vi "R5DOControl.vi"(8 "error constant":errorcluster, 11 "LabVIEW Web Service":refnum<class "Web Service.lvclass">) -> ()   [LabVIEW 2016]
uses:
  <vilib>/wsapi/Web Service.lvclass
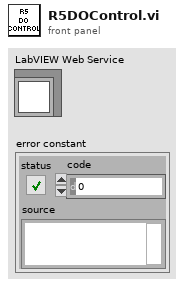
[diagram p1: front panel]
types:
  T1 = cluster{"Set Point, mg/L":dbl, "Tolerance, mg/L":dbl, "N2 Valve Gain":dbl, "Air Valve Gain":dbl}
  T2 = cluster{"Signal, mA":dbl, "Value, UNITS HERE":dbl}
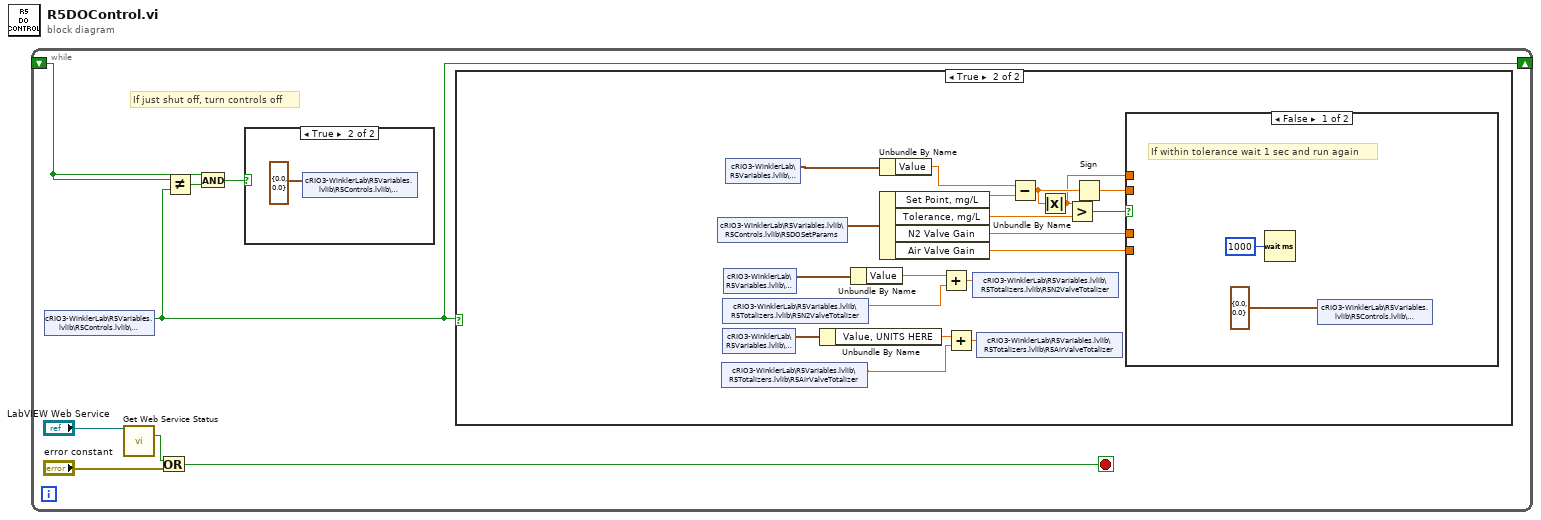
[diagram p0: block diagram]
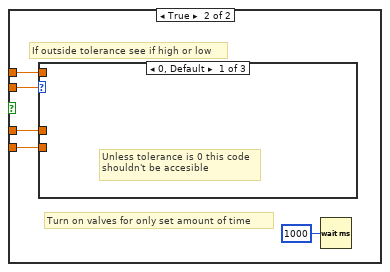
[diagram p4: hidden frame]
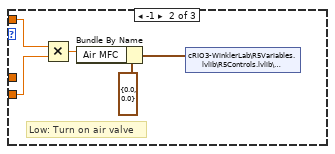
[diagram p5: hidden frame]
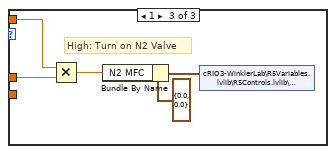
[diagram p6: hidden frame]
diagram:
  n1 = while {
    shift-right: [w1] -> _
    shift-left: _ -> [w2]
    stop <- w5 stop-if-true
    # "If just shut off, turn controls off"
    n2 = shared-variable "cRIO3-WinklerLab\\R5Variables.lvlib\\R5Controls.lvlib\\R5DOSwitch"() -> (w1:bool)  [unwired: 1 in, 1 out]
    n3 = call <vilib>:"Get Web Service Status.vi"("LabVIEW Web Service"="LabVIEW Web Service") -> ("service stopping?"=w8:bool)  [unwired: 12 in, 2 out]
    n4 = Or(x=w8, y="error constant") -> (x .or. y?=w5:bool)
    n5 = Not Equal?(x=w2, y=w1) -> (x != y?=w3:bool)
    n6 = And(x=w2, y=w3) -> (x .and. y?=w4:bool)
    n7 = case shown="True" w4 {
      frame False {
      }
      frame True {
        n8 = shared-variable "cRIO3-WinklerLab\\R5Variables.lvlib\\R5Controls.lvlib\\R5DOManual"(cluster{"Air MFC":dbl, "N2 MFC":dbl} {"Air MFC"=0.0, "N2 MFC"=0.0} ("R1DOManual")) -> ()  [unwired: 1 in, 1 out]
      }
    }
    n9 = case shown="True" w1 {
      frame False {
        # "Don't do anything if control is off"
      }
      frame True {
        n10 = shared-variable "cRIO3-WinklerLab\\R5Variables.lvlib\\R5Controls.lvlib\\R5DOSetParams"() -> (w16:T1)  [unwired: 1 in, 1 out]
        n11 = shared-variable "cRIO3-WinklerLab\\R5Variables.lvlib\\R5Totalizers.lvlib\\R5AirValveTotalizer"() -> (w13:dbl)  [unwired: 1 in, 1 out]
        n12 = shared-variable "cRIO3-WinklerLab\\R5Variables.lvlib\\R5Totalizers.lvlib\\R5N2ValveTotalizer"() -> (w12:dbl)  [unwired: 1 in, 1 out]
        n13 = shared-variable "cRIO3-WinklerLab\\R5Variables.lvlib\\R5Signals.lvlib\\R5Air"() -> (w14:T2)  [unwired: 1 in, 1 out]
        n14 = shared-variable "cRIO3-WinklerLab\\R5Variables.lvlib\\R5Signals.lvlib\\R5N2"() -> (w15:cluster{"Signal":dbl, "Value":dbl})  [unwired: 1 in, 1 out]
        n15 = shared-variable "cRIO3-WinklerLab\\R5Variables.lvlib\\R5Signals.lvlib\\R5DO"() -> (w17:cluster{"Signal":dbl, "Value":dbl})  [unwired: 1 in, 1 out]
        n16 = Unbundle By Name(w14) -> ("Value, UNITS HERE"=w19:dbl)
        n17 = Unbundle By Name(w15) -> ("Value"=w18:dbl)
        n18 = Unbundle By Name(w17) -> ("Value"=w28:dbl)
        n19 = Unbundle By Name(w16) -> ("Set Point, mg/L"=w27:dbl, "Tolerance, mg/L"=w26:dbl, "N2 Valve Gain"=w23:dbl, "Air Valve Gain"=w22:dbl)
        n20 = Add(x=w18, y=w12) -> (x+y=w11:dbl)
        n21 = Add(x=w19, y=w13) -> (x+y=w10:dbl)
        n22 = shared-variable "cRIO3-WinklerLab\\R5Variables.lvlib\\R5Totalizers.lvlib\\R5N2ValveTotalizer"(w11) -> ()  [unwired: 1 in, 1 out]
        n23 = shared-variable "cRIO3-WinklerLab\\R5Variables.lvlib\\R5Totalizers.lvlib\\R5AirValveTotalizer"(w10) -> ()  [unwired: 1 in, 1 out]
        n24 = Subtract(x=w28, y=w27) -> (x-y=w21:dbl)
        n25 = Absolute Value(x=w21) -> (abs(x)=w20:dbl)
        n26 = Greater?(x=w20, y=w26) -> (0:w25:bool)
        n27 = Sign(1:w21) -> (0:w24:dbl)
        n28 = case shown="False" w25 {
          tunnel: w24 -> [_ w35]
          tunnel: w23 -> [_ w34]
          tunnel: w22 -> [_ w33]
          tunnel: w20 -> [_ w32]
          frame False {
            # "If within tolerance wait 1 sec and run again"
            n29 = Wait (ms)(milliseconds to wait=u32 1000) -> ()  [unwired: 1 out]
            n30 = shared-variable "cRIO3-WinklerLab\\R5Variables.lvlib\\R5Controls.lvlib\\R5DOManual"(cluster{"Air MFC":dbl, "N2 MFC":dbl} {"Air MFC"=0.0, "N2 MFC"=0.0} ("R1DOManual")) -> ()  [unwired: 1 in, 1 out]
          }
          frame True {
            # "Turn on valves for only set amount of time"
            # "If outside tolerance see if high or low"
            n31 = case shown="0, Default" w35 {
              tunnel: w33 -> [_ w37 _]
              tunnel: w34 -> [_ _ w43]
              tunnel: w32 -> [_ w38 w44]
              frame 0, Default {
                # "Unless tolerance is 0 this code\nshouldn't be accesible"
              }
              frame -1 {
                # "Low: Turn on air valve"
                n32 = Multiply(x=w38, y=w37) -> (x*y=w39:dbl)
                n33 = Bundle By Name(cluster=cluster{"Air MFC":dbl, "N2 MFC":dbl} {"Air MFC"=0.0, "N2 MFC"=0.0} ("R1DOManual"), "Air MFC"=w39) -> (w36:cluster{"Air MFC":dbl, "N2 MFC":dbl})
                n34 = shared-variable "cRIO3-WinklerLab\\R5Variables.lvlib\\R5Controls.lvlib\\R5DOManual"(w36) -> ()  [unwired: 1 in, 1 out]
              }
              frame 1 {
                # "High: Turn on N2 Valve"
                n35 = Multiply(x=w44, y=w43) -> (x*y=w42:dbl)
                n36 = Bundle By Name(cluster=cluster{"Air MFC":dbl, "N2 MFC":dbl} {"Air MFC"=0.0, "N2 MFC"=0.0} ("R1DOManual"), "N2 MFC"=w42) -> (w41:cluster{"Air MFC":dbl, "N2 MFC":dbl})
                n37 = shared-variable "cRIO3-WinklerLab\\R5Variables.lvlib\\R5Controls.lvlib\\R5DOManual"(w41) -> ()  [unwired: 1 in, 1 out]
              }
            }
            n38 = Wait (ms)(milliseconds to wait=u32 1000) -> ()  [unwired: 1 out]
          }
        }
      }
    }
  }
